vi "CreateTopic.vi"(8 "error in (no error)":errorcluster, 9 "1:M":bool, 10 "Topic Name":string, 11 "Websocket Message Broker in":refnum<class "Websocket Message Broker.lvclass">) -> (0 "error out":errorcluster, 2 "Locked?":bool, 3 "Websocket Message Broker out":refnum<class "Websocket Message Broker.lvclass">, 5 "Transport":refnum<class "Message Transport Queue.lvclass">)   [LabVIEW 2016, in "Stream Mediator.lvlib" / "Websocket Message Broker.lvclass"]
doc: "--\nCopyright © 2017 Composed SystemsI All rights reserved.\n\nAuthor: Jon McBee <jon.mcbee@composed.io>\n\nThis library is provided \"AS IS\" ,WITHOUT WARRANTIES OR\nCONDITIONS OF ANY KIND, either express or implied.\n\nComposed Systems -- composed.io\n\nStream 0.0.1.1\nJon McBee - Composed Systems\nCopyright (c) 2017, Composed Systems"
uses:
  <userlib>/Composed Systems/Stream/Mediator/Classes/Websocket Message Broker/Websocket Message Broker.lvclass
  <userlib>/Composed Systems/Stream/Mediator/Classes/Message Transport Queue/Message Transport Queue.lvclass
  <userlib>/Composed Systems/Stream/Mediator/Classes/Message Broker/Message Broker.lvclass
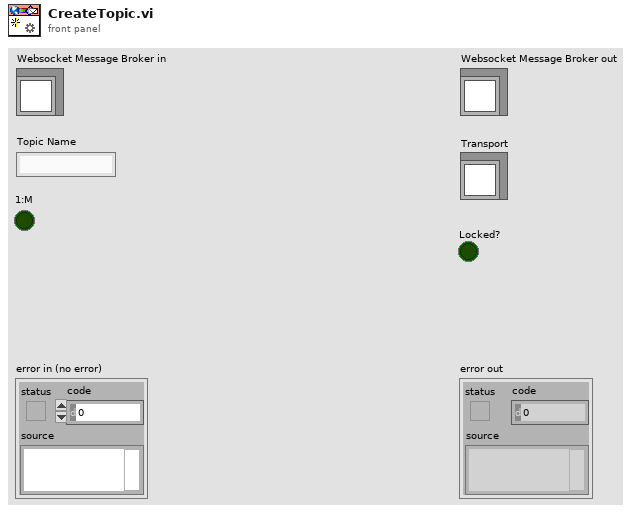
[diagram p1: front panel]
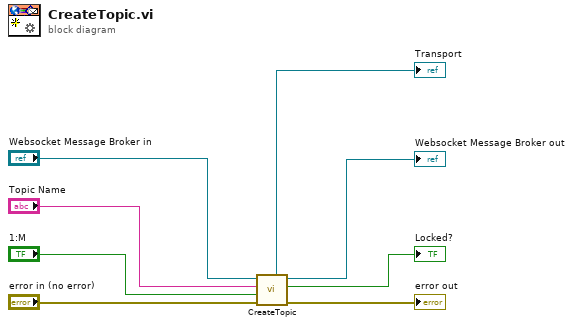
[diagram p0: block diagram]
diagram:
  n1 = call-parent "CreateTopic.vi"("error in (no error)"="error in (no error)", "1:M"="1:M", "Topic Name"="Topic Name", "Message Broker in"="Websocket Message Broker in") -> ("error out"=→"error out":errorcluster, "Locked?"=→"Locked?":bool, "Message Broker out"=→"Websocket Message Broker out":refnum<class "Websocket Message Broker.lvclass">, "Transport"=→"Transport":refnum<class "Message Transport Queue.lvclass">)  [unwired: 4 in]
